vi "Exemple_Preprocessing_label_binarize.vi"() -> ()   [LabVIEW 2020]
panel:
  out "Data":T1
  out "error out":errorcluster
  in  "y":string[][](array[string])=[["1", "6"]]
  in  "error in":errorcluster caption="entrée d'erreur"
  in  "label_binarize":T2={"classes"=[["1"], ["2"], ["4"], ["6"]], "neg_label"=0, "pos_label"=1, "sparse_output"=FALSE}
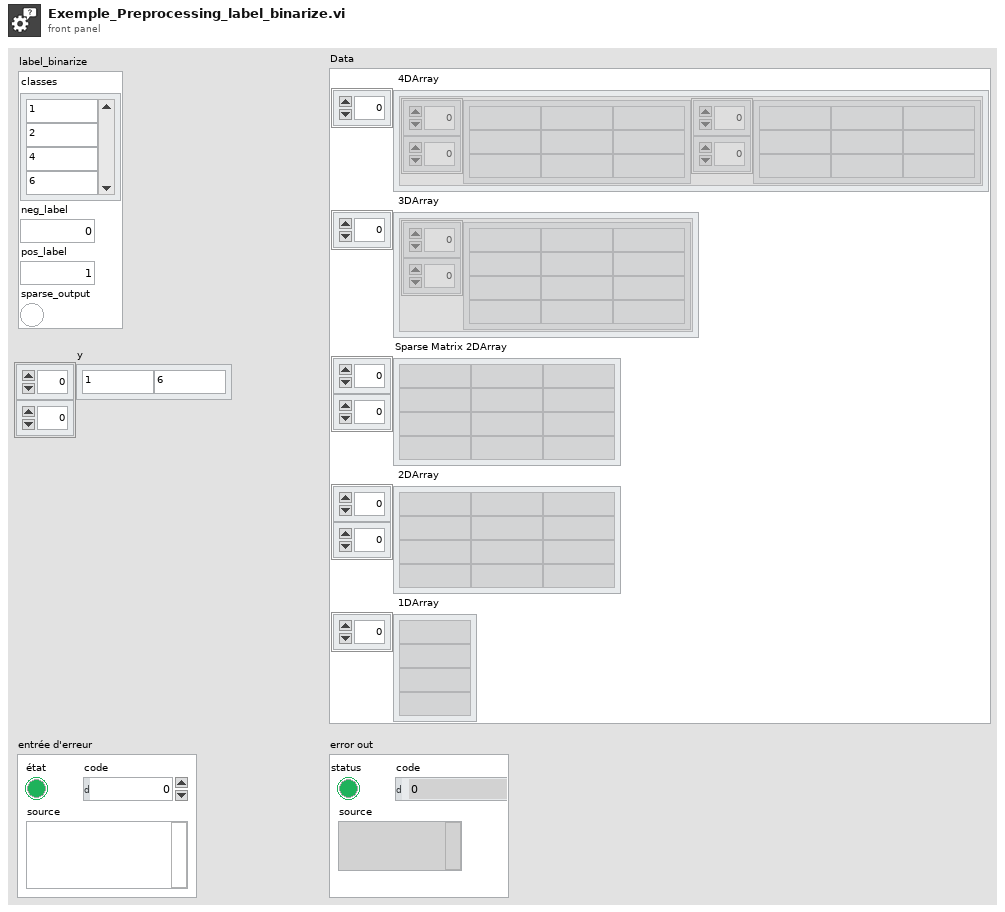
[diagram p1: front panel]
types:
  T1 = cluster{" 4DArray":cluster{"1":string[][], "2":string[][]}[], " 3DArray":cluster{"Tableau":string[][]}[], "Sparse Matrix 2DArray":string[][], " 2DArray":string[][], " 1DArray":string[]}
  T2 = cluster{"classes":string[][], "neg_label":i32, "pos_label":i32, "sparse_output":bool}
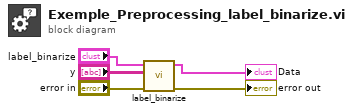
[diagram p0: block diagram]
diagram:
  n1 = call "label_binarize.vi"("error in"="error in", "y"="y", "label_binarize"="label_binarize") -> ("error out"=→"error out":errorcluster, "Data"=→"Data":T1)  [unwired: 7 in]
